vi "DMR_GetImageRequestBufferImageData.vi"(0 "driver handle IN":u32, 1 "request number IN":u32, 2 "bytes per pixel IN":u32, 4 "X-offset IN":u32, 5 "Y-offset IN":u32, 7 "height IN":u32, 9 "width IN":u32) -> (14 "driver handle OUT":u32, 15 "request number OUT":u32, 17 "image OUT":u32[][](array[numeric]), 19 "error code OUT":i32)   [LabVIEW 2014]
doc: "Returns an AOI of raw image data belonging to the specified request.\n\nThe 'request number IN' parameter can be obtained from the DMR_ImageRequestWaitFor VI.\n\nPlease note, that the usage of the sub-VIs called by this VI (e.g. 'DMR_GetImageRequestBufferImageData8Bit') perform much more efficient as no data conversion has to be performed within LabVIEW. For applications with known pixel formats therefore these VIs should be used.\n\nSee also:\nDMR_GetImageRequestBufferChannelData\n\nThe 'error code OUT' terminal will deliver 0 if successful or a negative error code otherwise. A list of valid error codes and their meaning can be found in the manual about this interface."
panel:
  # "OUTPUT"
  # "INPUT"
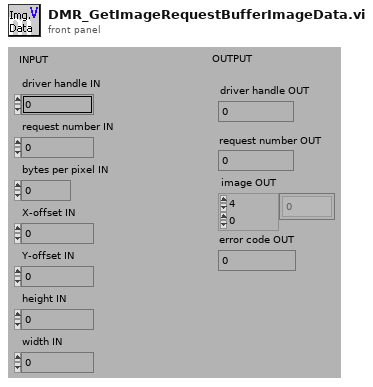
[diagram p1: front panel]
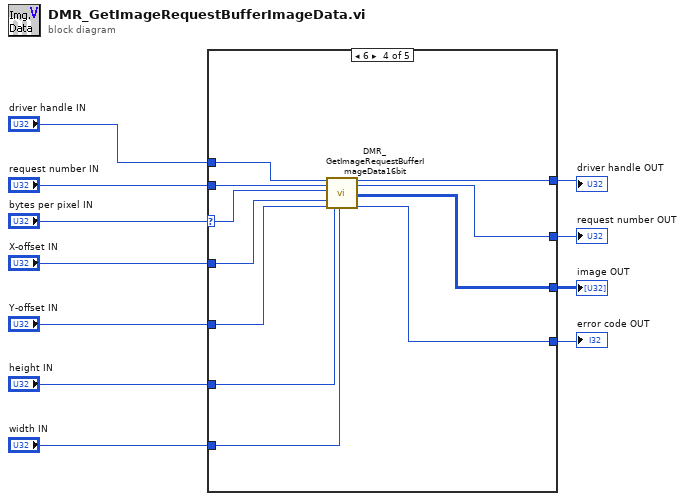
[diagram p0: block diagram]
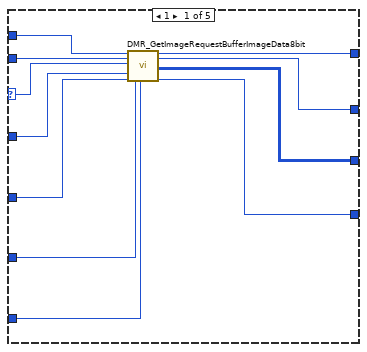
[diagram p2: hidden frame]
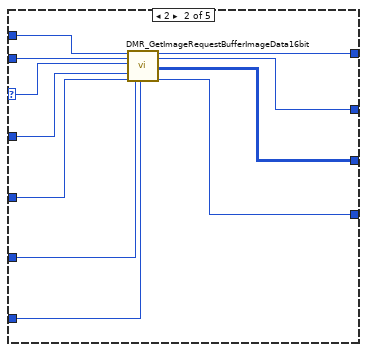
[diagram p3: hidden frame]
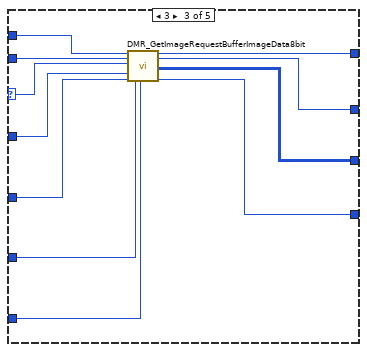
[diagram p4: hidden frame]
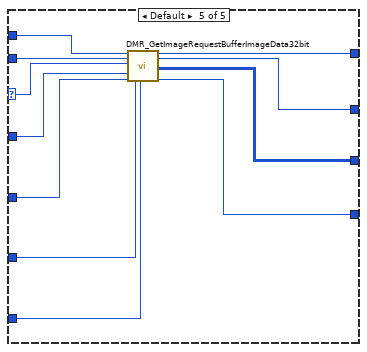
[diagram p5: hidden frame]
diagram:
  n1 = case shown="6" "bytes per pixel IN" {
    selector: "bytes per pixel IN" -> [w12 w23 w34 w45 w56]
    tunnel: "driver handle IN" -> [w22 w33 w44 w55 w66]
    tunnel: "request number IN" -> [w21 w32 w43 w54 w65]
    tunnel: "X-offset IN" -> [w20 w31 w42 w53 w64]
    tunnel: "Y-offset IN" -> [w19 w30 w41 w52 w63]
    tunnel: "height IN" -> [w18 w29 w40 w51 w62]
    tunnel: [w17 w27 w39 w49 w60] -> w5
    tunnel: [w16 w24 w38 w46 w57] -> w4
    tunnel: "width IN" -> [w15 w28 w37 w50 w61]
    tunnel: [w14 w26 w36 w48 w59] -> w2
    tunnel: [w13 w25 w35 w47 w58] -> w1
    frame 1 {
      n2 = call "DMR_GetImageRequestBufferImageData8bit.vi"("driver handle IN"=w22, "request number IN"=w21, "bytes per pixel IN"=w12, "X-offset"=w20, "Y-offset"=w19, "height"=w18, "width"=w15) -> ("driver handle OUT"=w17:u32, "request number OUT"=w14:u32, "image OUT"=w13:u8[][], "error code OUT"=w16:i32)  [unwired: 9 in]
    }
    frame 2 {
      n3 = call "DMR_GetImageRequestBufferImageData16bit.vi"("driver handle IN"=w33, "request number IN"=w32, "bytes per pixel IN"=w23, "X-offset"=w31, "Y-offset"=w30, "height"=w29, "width"=w28) -> ("driver handle OUT"=w27:u32, "request number OUT"=w26:u32, "image OUT"=w25:u16[][], "error code OUT"=w24:i32)  [unwired: 9 in]
    }
    frame 3 {
      n4 = call "DMR_GetImageRequestBufferImageData8bit.vi"("driver handle IN"=w44, "request number IN"=w43, "bytes per pixel IN"=w34, "X-offset"=w42, "Y-offset"=w41, "height"=w40, "width"=w37) -> ("driver handle OUT"=w39:u32, "request number OUT"=w36:u32, "image OUT"=w35:u8[][], "error code OUT"=w38:i32)  [unwired: 9 in]
    }
    frame 6 {
      n5 = call "DMR_GetImageRequestBufferImageData16bit.vi"("driver handle IN"=w55, "request number IN"=w54, "bytes per pixel IN"=w45, "X-offset"=w53, "Y-offset"=w52, "height"=w51, "width"=w50) -> ("driver handle OUT"=w49:u32, "request number OUT"=w48:u32, "image OUT"=w47:u16[][], "error code OUT"=w46:i32)  [unwired: 9 in]
    }
    frame Default {
      n6 = call "DMR_GetImageRequestBufferImageData32bit.vi"("driver handle IN"=w66, "request number IN"=w65, "bytes per pixel IN"=w56, "X-offset"=w64, "Y-offset"=w63, "height"=w62, "width"=w61) -> ("driver handle OUT"=w60:u32, "request number OUT"=w59:u32, "image OUT"=w58:u32[][], "error code OUT"=w57:i32)  [unwired: 9 in]
    }
  }
  "error code OUT" <- w4
  "request number OUT" <- w2
  "image OUT" <- w1
  "driver handle OUT" <- w5
